vi "receive header message.vi"(8 "error in (no error)":errorcluster, 11 "Channel in":refnum<class "Channel.lvclass">) -> (0 "error out":errorcluster, 3 "Channel out":refnum<class "Channel.lvclass">)   [LabVIEW 2018, in "Channel.lvclass"]
uses:
  Channel.lvclass
  Channel.lvclass/Channel.ctl
  Header content/Header content.lvclass
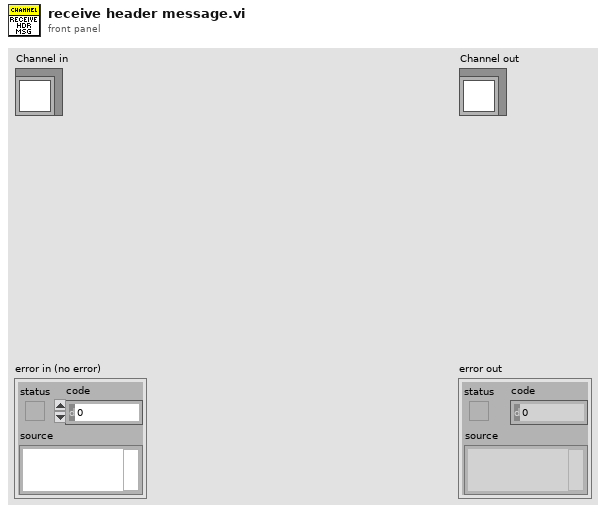
[diagram p1: front panel]
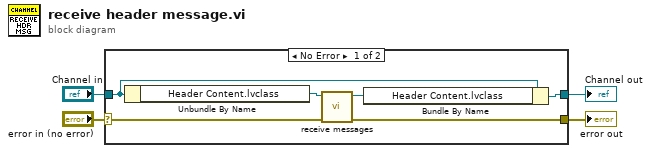
[diagram p0: block diagram]
diagram:
  n1 = case shown="No Error" "error in (no error)" {
    selector: "error in (no error)" -> [w9 w12]
    tunnel: [w5 w12] -> w3
    tunnel: [w7 w11] -> w1
    tunnel: "Channel in" -> [w8 w11]
    frame No Error {
      n2 = Unbundle By Name(w8) -> ("Header Content.lvclass"=w10:refnum<class "Header content.lvclass">)
      n3 = call "receive messages.vi"("error in (no error)"=w9, "Header content in"=w10) -> ("error out"=w5:errorcluster, "Header content out"=w6:refnum<class "Header content.lvclass">)  [unwired: 8 in]
      n4 = Bundle By Name(cluster=w8, "Header Content.lvclass"=w6) -> (w7:refnum<class "Channel.lvclass">)
    }
    frame Error {
    }
  }
  "error out" <- w3
  "Channel out" <- w1
